vi "Button Reset.vi"(8 "error in (no error)":errorcluster, 11 "State Data in":T1) -> (0 "error out":errorcluster, 3 "State Data out":T1)   [LabVIEW 2025]
uses:
  State Data.ctl
  Team.ctl
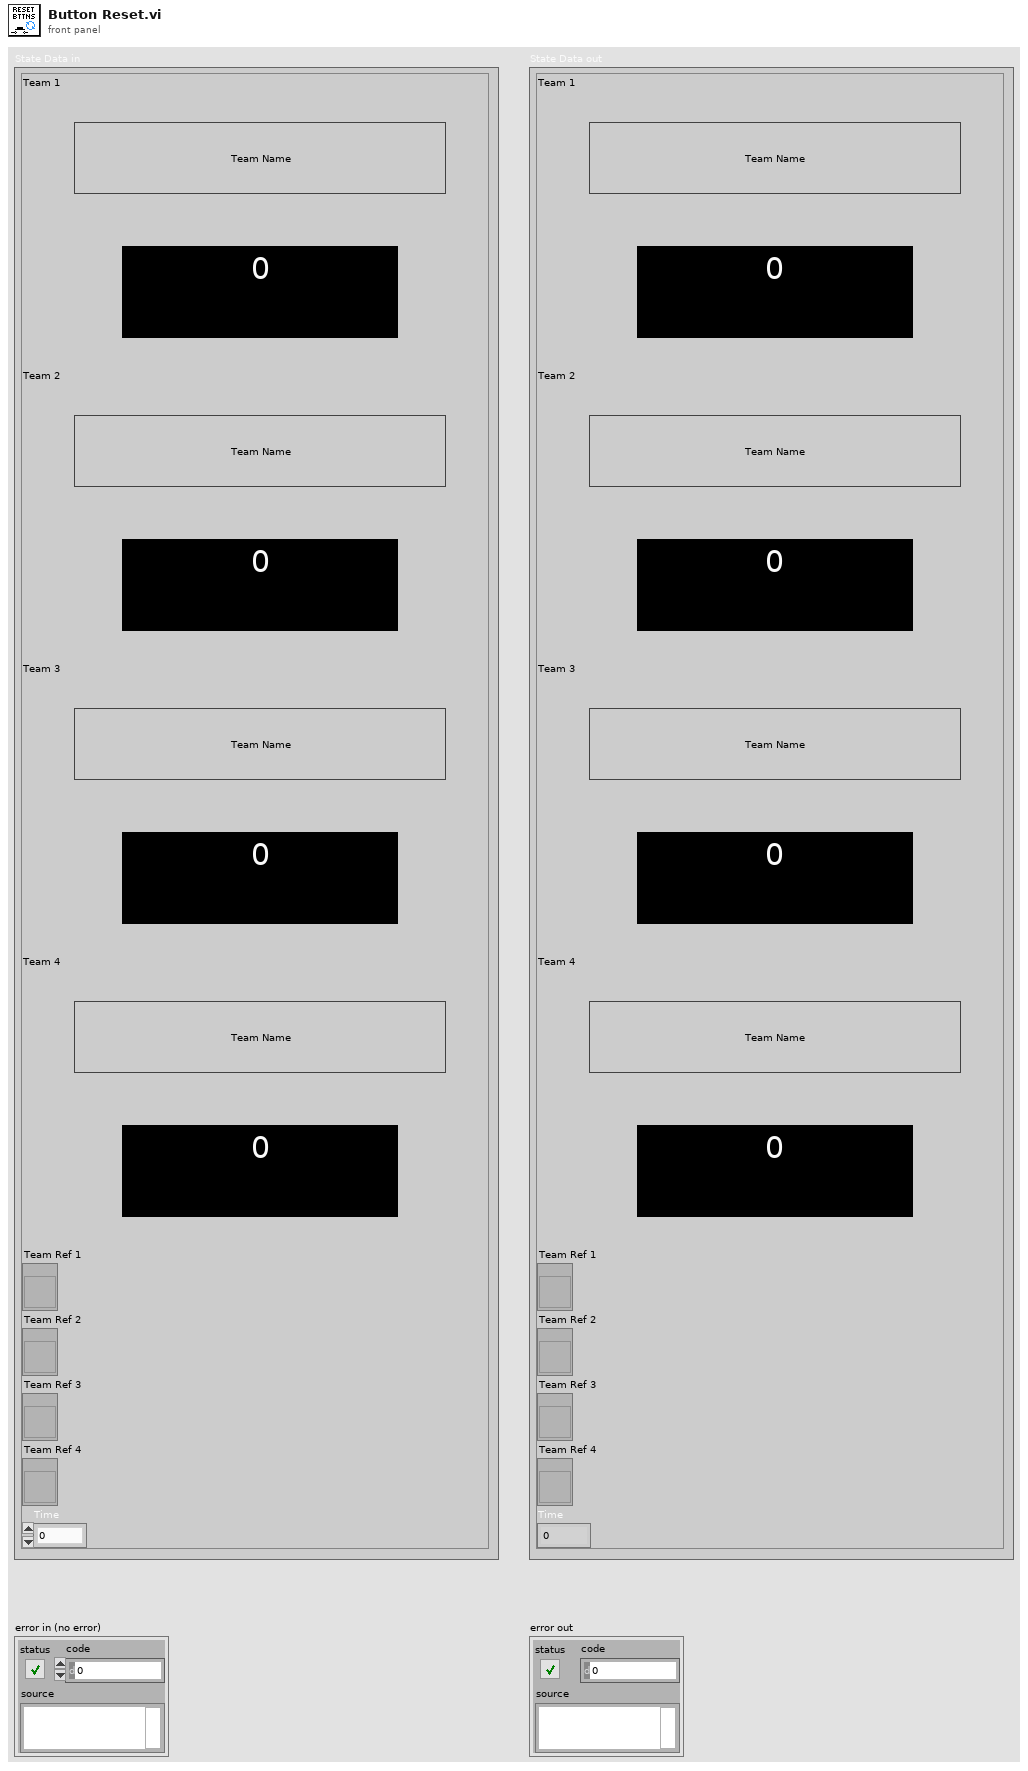
[diagram p1: front panel]
types:
  T1 = typedef "State Data.ctl" = cluster{"Team 1":T2, "Team 2":T2, "Team 3":T2, "Team 4":T2, "Team Ref 1":refnum<vi>, "Team Ref 2":refnum<vi>, "Team Ref 3":refnum<vi>, "Team Ref 4":refnum<vi>, "Time":i32}
  T2 = typedef "Team.ctl" = cluster{"ON":bool, "Name":bool, "Score":i32, "Split":string}
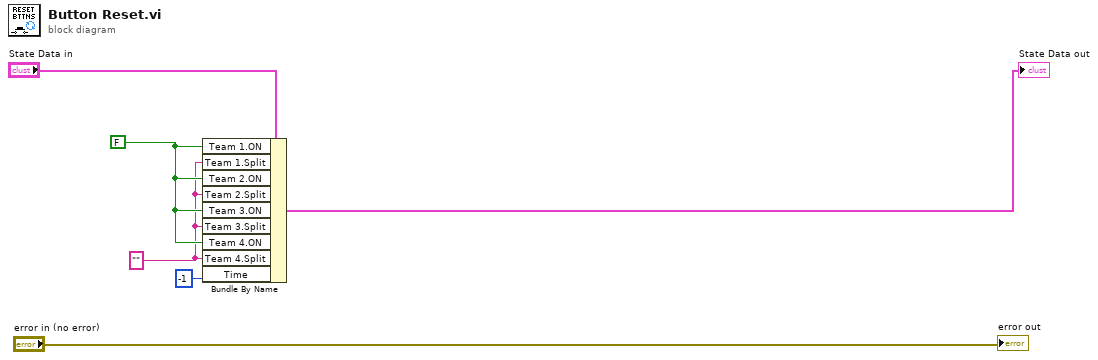
[diagram p0: block diagram]
diagram:
  w1 = "" ("Team 1.Split")
  w2 = FALSE ("Team 1.ON")
  n1 = Bundle By Name(cluster="State Data in", "Team 1.ON"=w2, "Team 1.Split"=w1, "Team 2.ON"=w2, "Team 2.Split"=w1, "Team 3.ON"=w2, "Team 3.Split"=w1, "Team 4.ON"=w2, "Team 4.Split"=w1, "Time"=-1) -> (→"State Data out":T1)
  "error out" <- "error in (no error)"
